vi "patientTrainingView.vi"() -> ()   [LabVIEW 2019]
doc: "40"
uses:
  03_Home/controller/logoutBtn.ctl
  03_Home/controller/exitBtn.ctl
  <vilib>/Utility/miscctls.llb/LVPointTypeDef.ctl
  subVI/patients_state.ctl
  <vilib>/Utility/miscctls.llb/LVSelectionTypeDef.ctl
  03_Home/controller/pannelState.ctl
  globalValue.vi
panel:
  out "patients_nm2":string
  out "training_id":string[](array[string])
  out "totalCount":string
  out "patients_info":string
  out "patients_notes":string
  out "patients_nm":string
  out "patients_id":string
  in  "patients_weight":dbl format="%.1f kg"
  in  "patients_age":dbl
  in  "patients_height":dbl format="%.1f cm"
  out "patients_birthdate":dbl format="%<%Y.%m.%d.>T"
  in  "backPage":bool
  in  "btnGroup":T1
  out "totalPage":i8
  out "crrentPage":i8
  in  "leftBtn":bool
  in  "rightBtn":bool
  in  "patientList":i32(listbox)
  in  "cancelBtn":bool
  in  "updateBtn":bool
  in  "deleteBtn":bool
  out "userDetailInfo":string[](array[string])
  in  "Help Button":bool
  in  "LogOut Button":T2
  in  "Exit Button":T3
  out "userNm":string
  # "/"
  # "|"
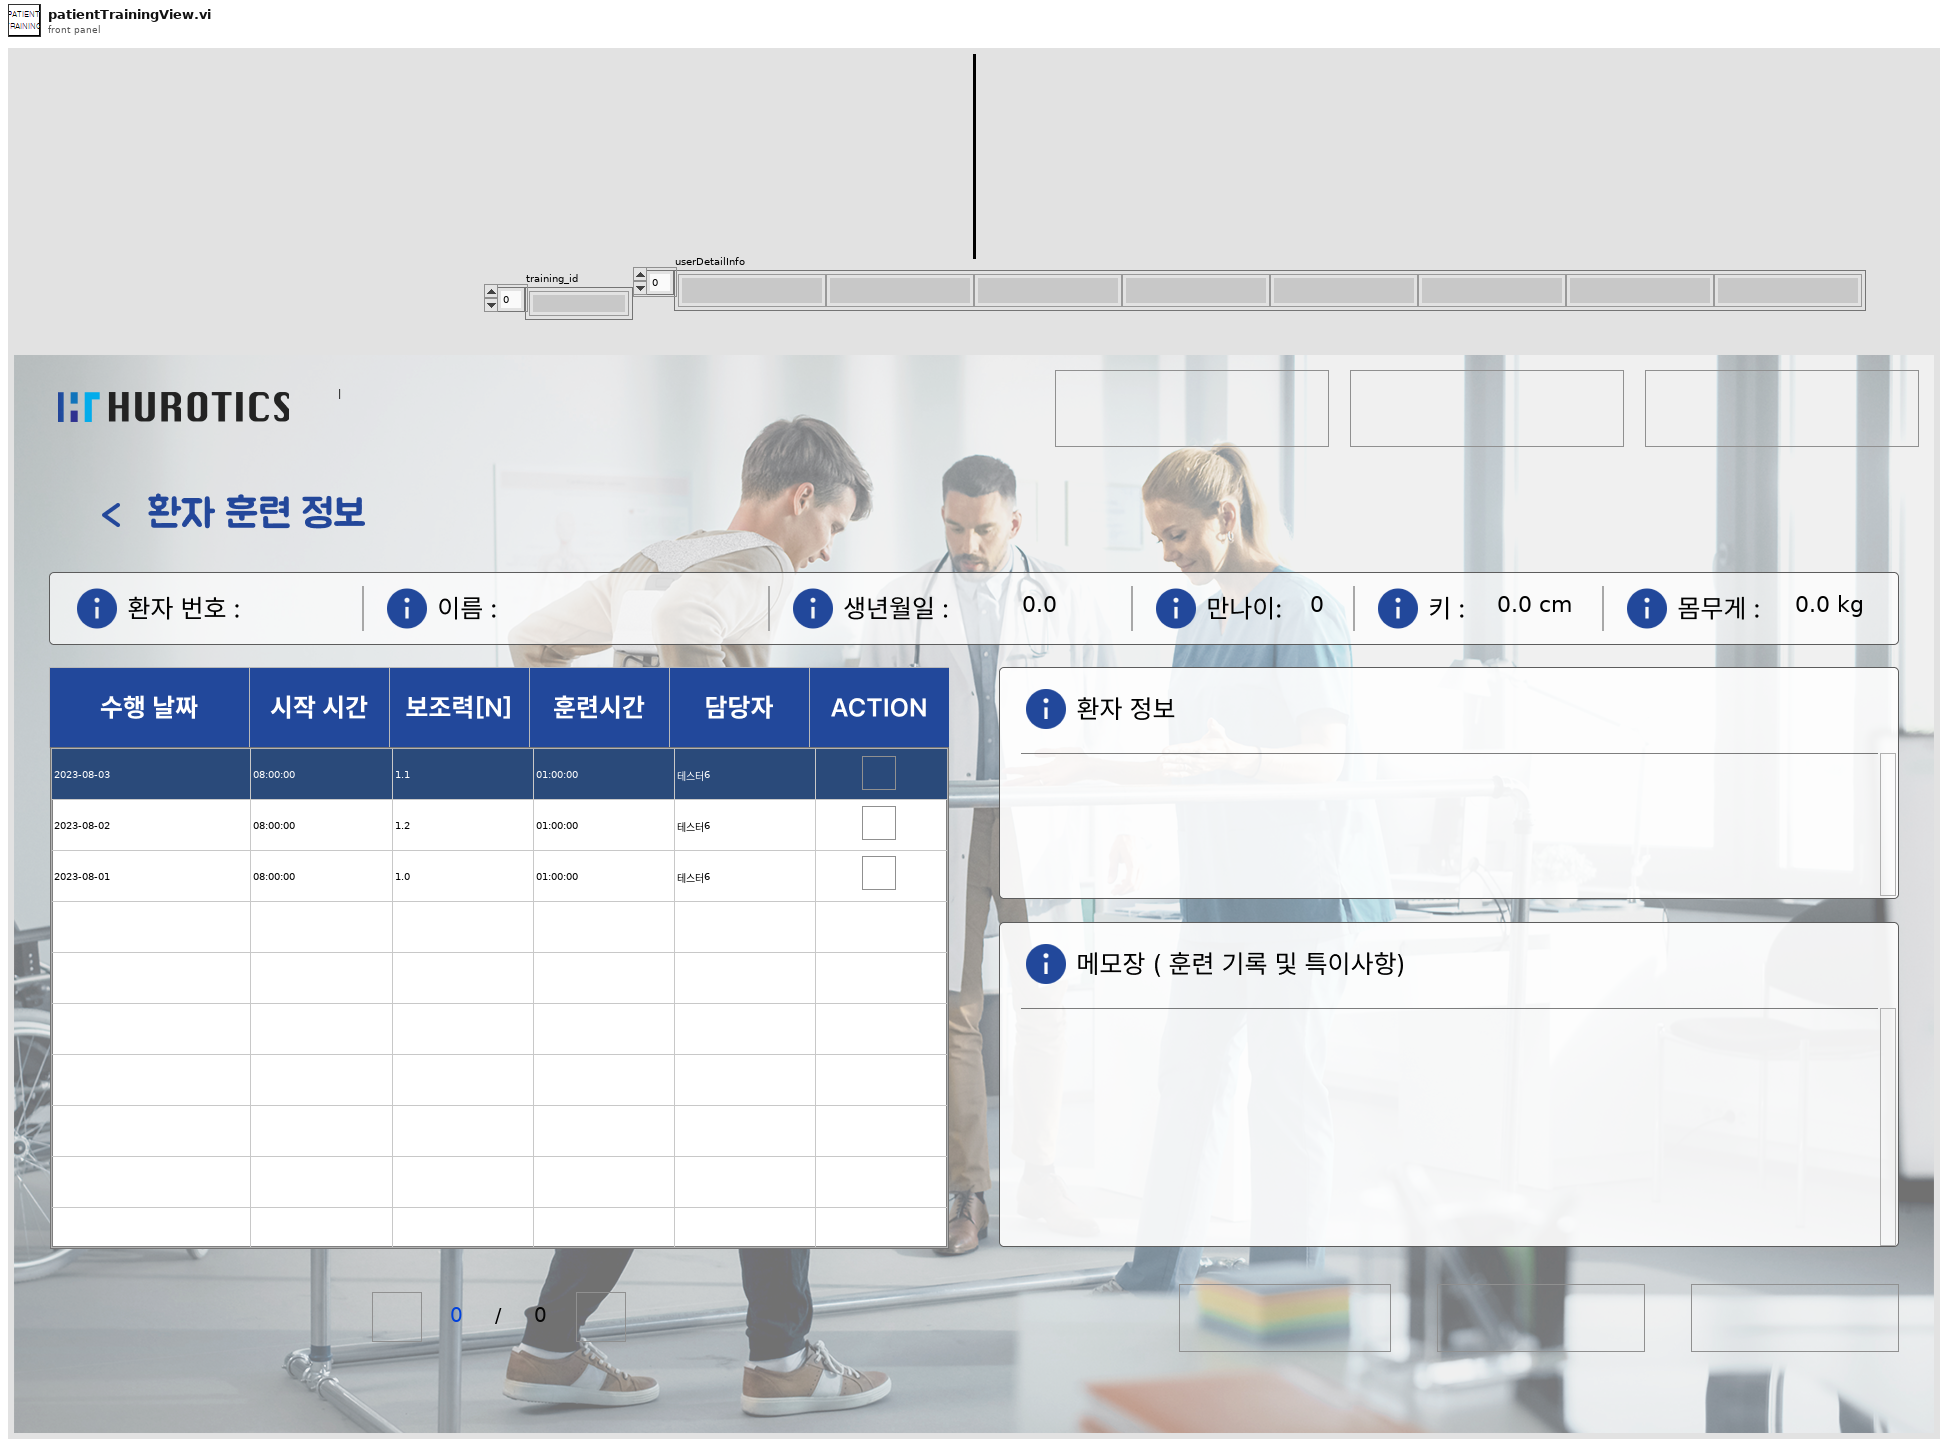
[diagram p1: front panel]
types:
  T1 = cluster{"detailBtn":bool, "detailBtn":bool, "detailBtn 2":bool, "detailBtn 3":bool, "detailBtn 4":bool, "detailBtn 5":bool, "detailBtn 6":bool, "detailBtn 7":bool, "detailBtn 8":bool, "detailBtn 9":bool}
  T2 = typedef "logoutBtn.ctl" = bool
  T3 = typedef "exitBtn.ctl" = bool
  T4 = typedef "LVPointTypeDef.ctl" = cluster{"Horizontal":i16, "Vertical":i16}
  T5 = typedef "patients_state.ctl" = enum16{"connection", "create", "getReadList", "getRead", "getCount", "update", "delete", "trash", "restore", "close"}
  T6 = enum16{"connection", "create", "getReadList", "getRead", "getCount", "update", "delete", "close"}
  T7 = typedef "LVSelectionTypeDef.ctl" = cluster{"Selection Start":u32, "Selection End":u32}
  T8 = enum8{"Enabled", "Disabled", "Disabled and Grayed Out"}
  T9 = typedef "pannelState.ctl" = enum16{"Init", "LogIn", "SignUpView", "Home", "Management_patientList", "Management_patientTrashtList", "Management_patientCreate", "Management_patientUpdate", "Management_patientTraining", "Management_patientTrainingDetail", "H-MEDI PatientList", "H-MEDI HardwareCtl", "Adjust", "FineTuning", "UserList", "UserDetail", "Exit"}
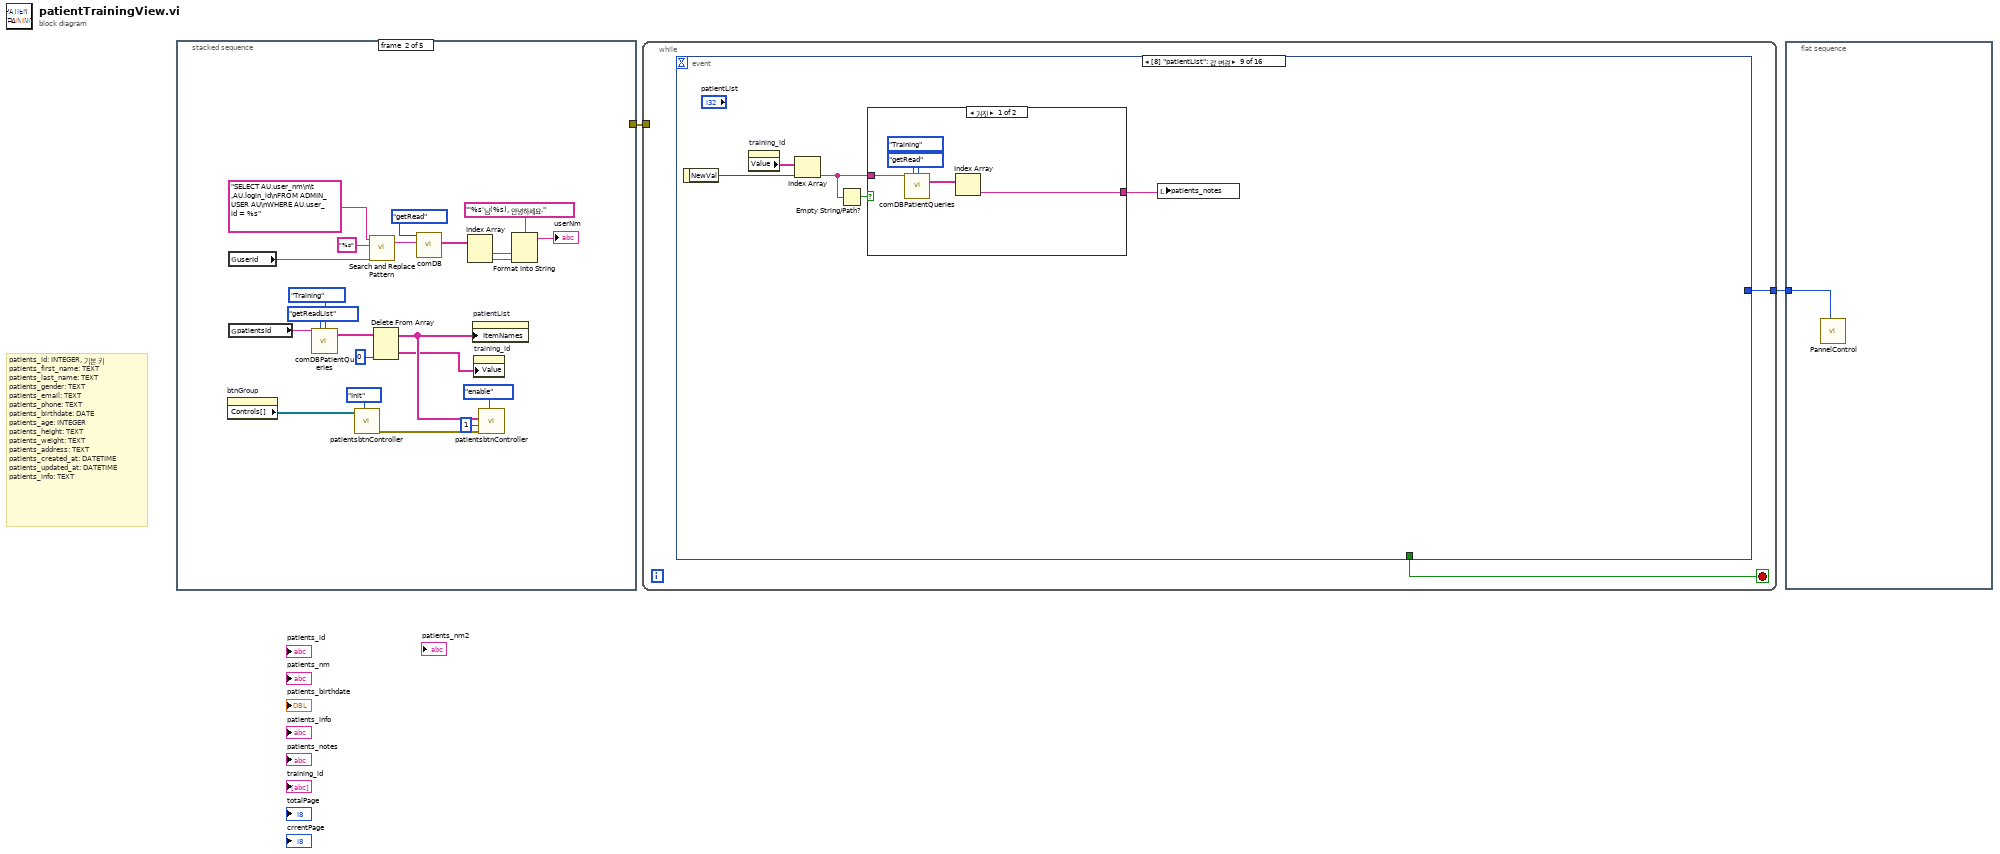
[diagram p0: block diagram]
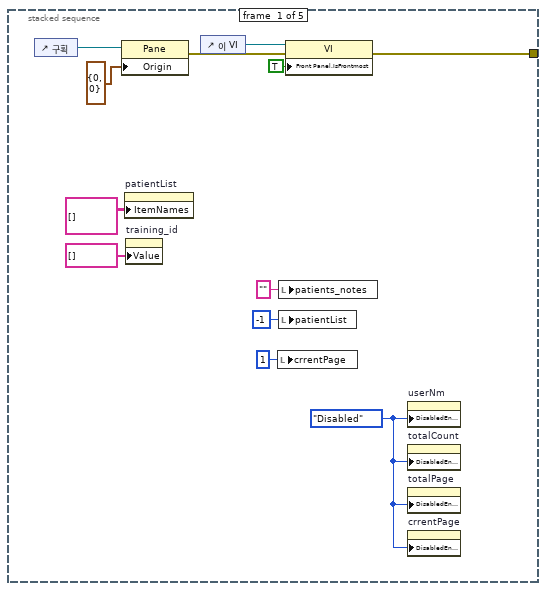
[diagram p2: hidden frame]
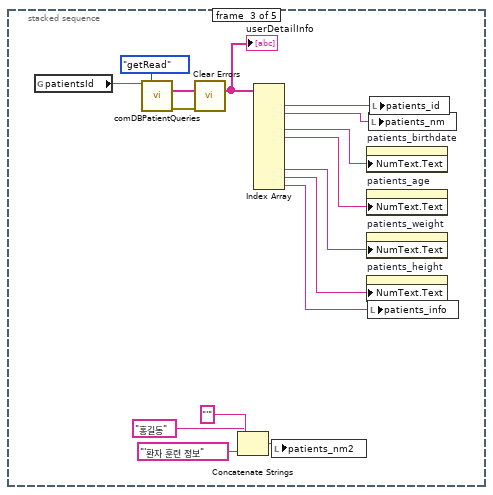
[diagram p3: hidden frame]
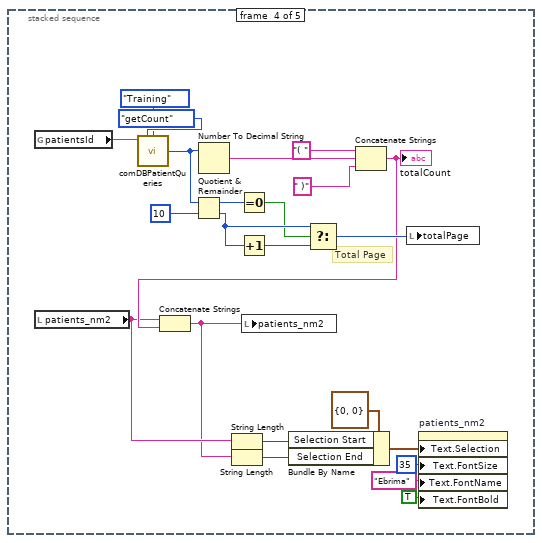
[diagram p4: hidden frame]
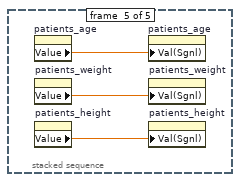
[diagram p5: hidden frame]
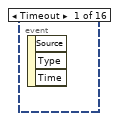
[diagram p6: hidden frame]
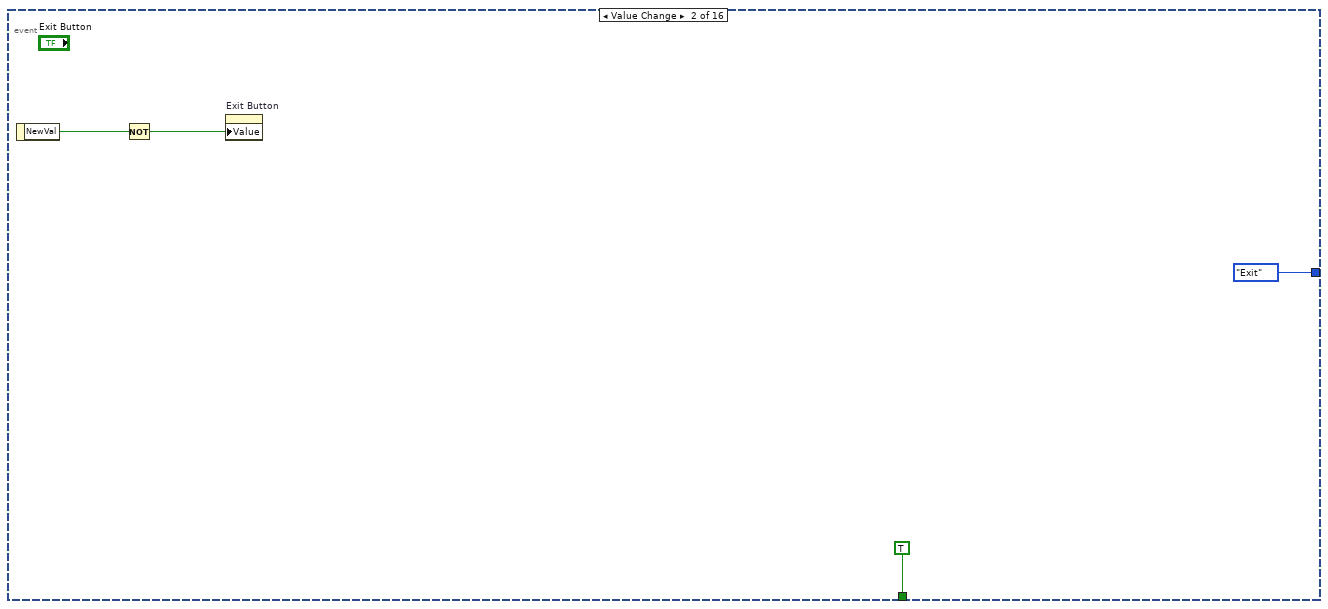
[diagram p7: hidden frame]
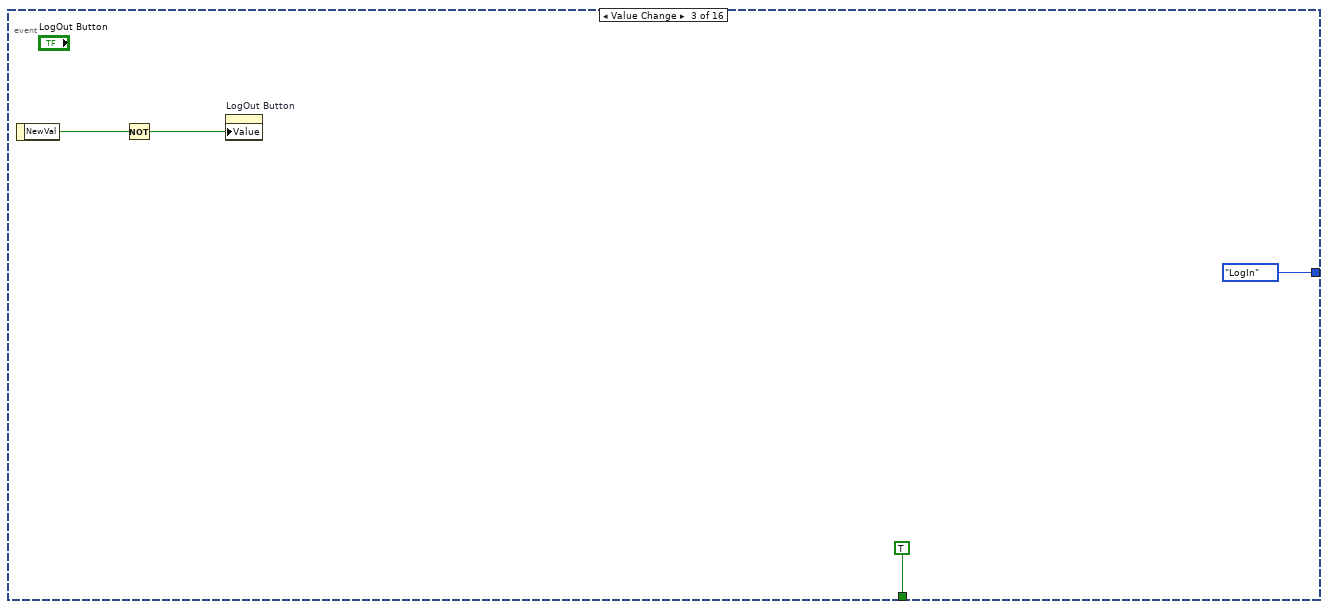
[diagram p8: hidden frame]
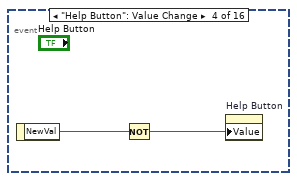
[diagram p9: hidden frame]
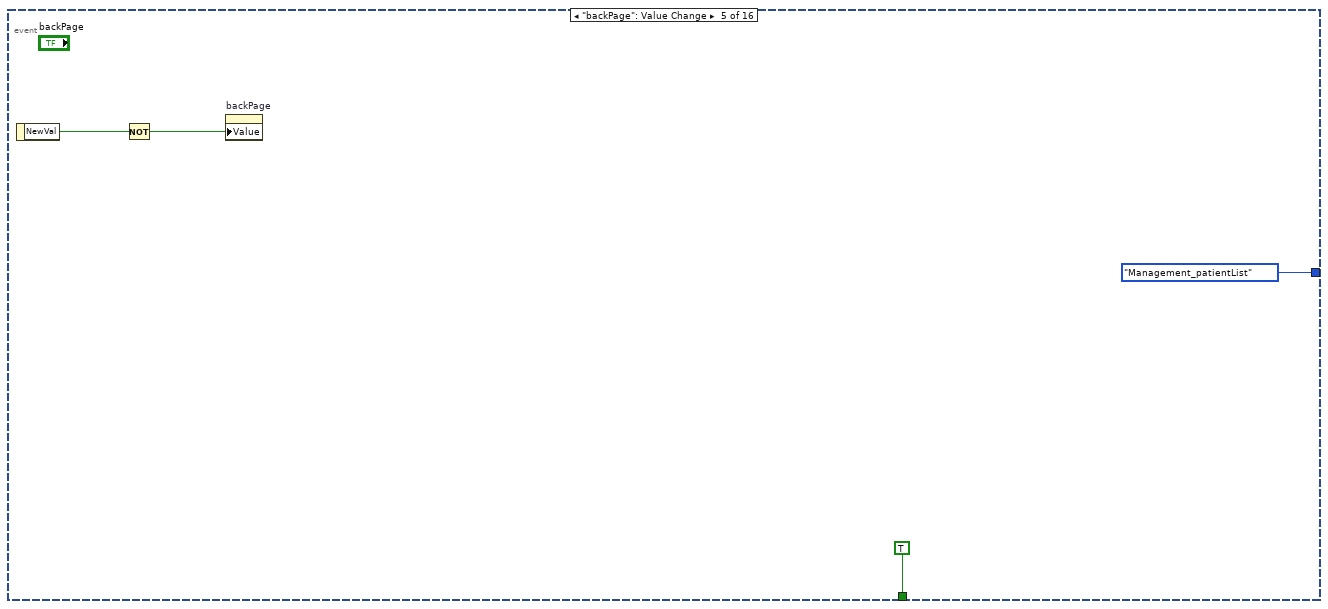
[diagram p10: hidden frame]
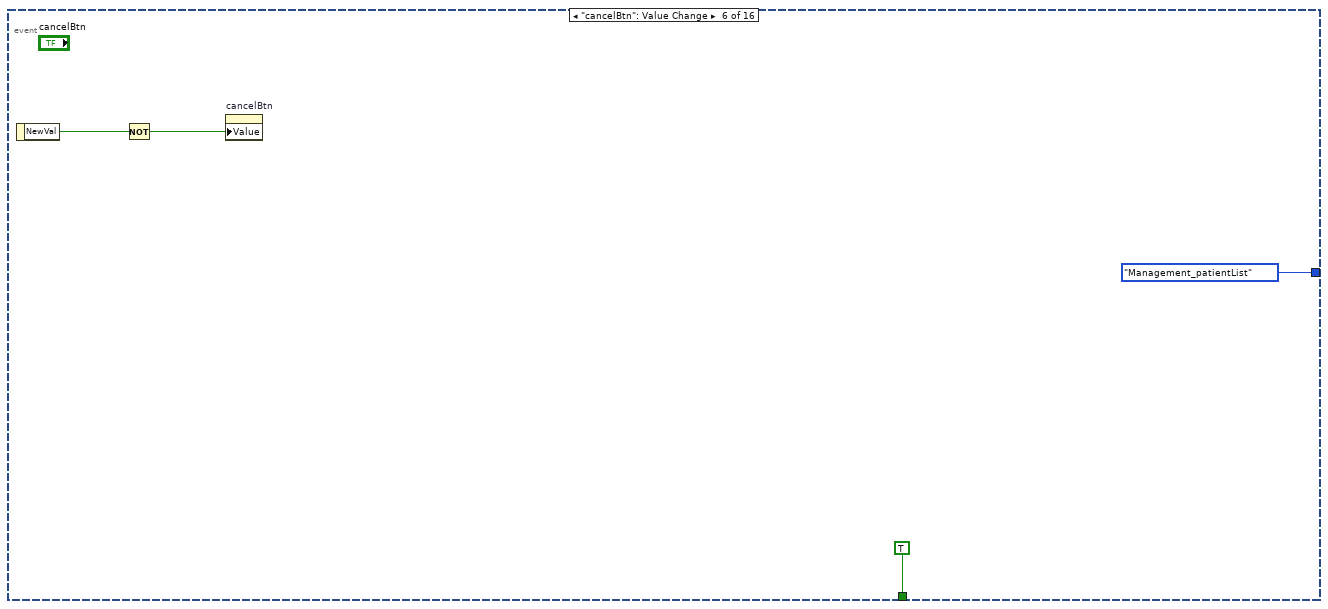
[diagram p11: hidden frame]
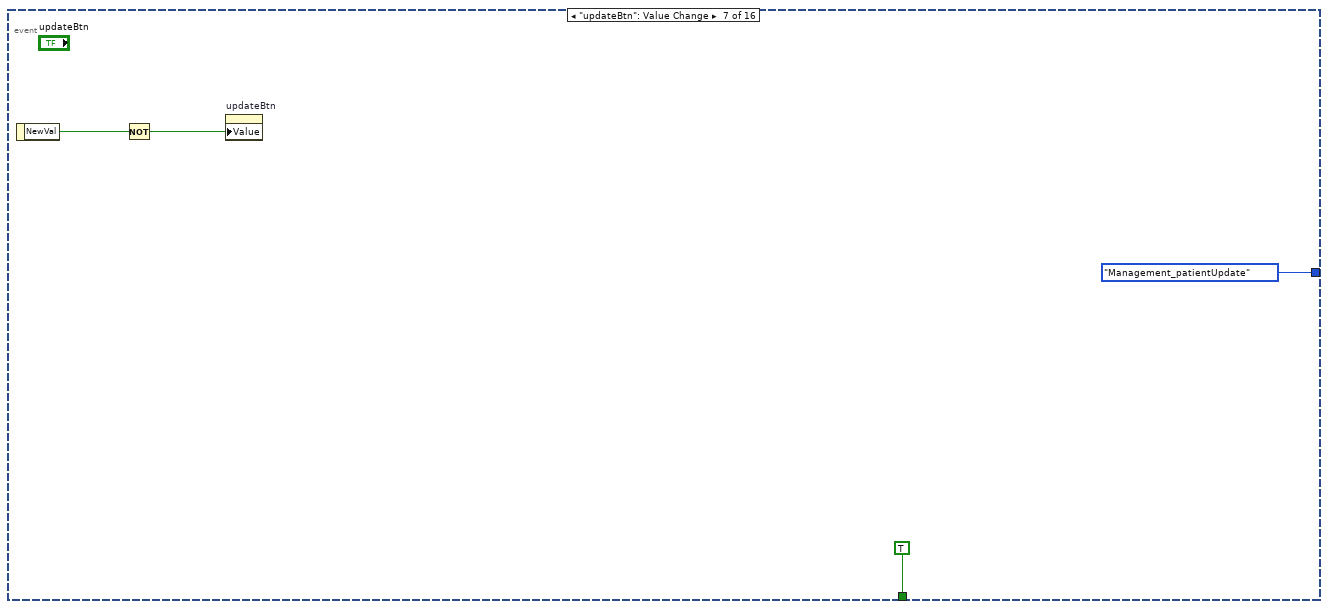
[diagram p12: hidden frame]
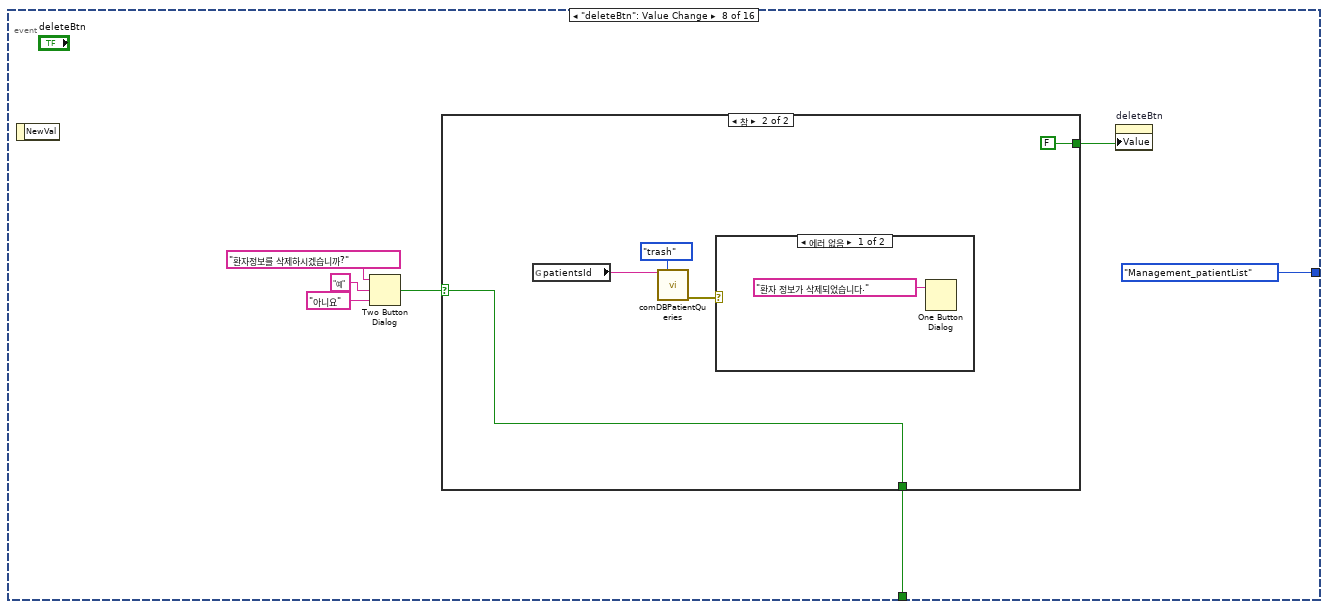
[diagram p13: hidden frame]
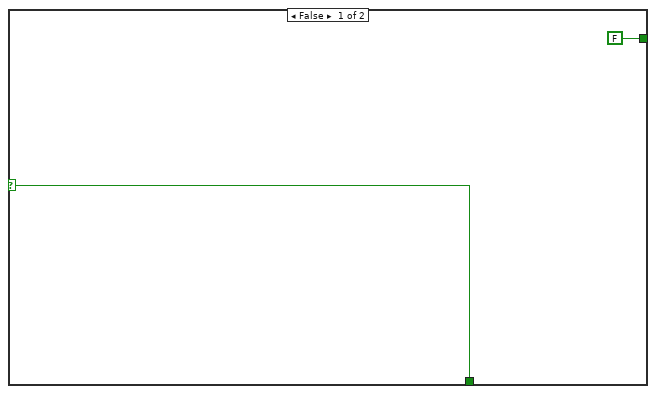
[diagram p14: hidden frame]
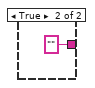
[diagram p16: hidden frame]
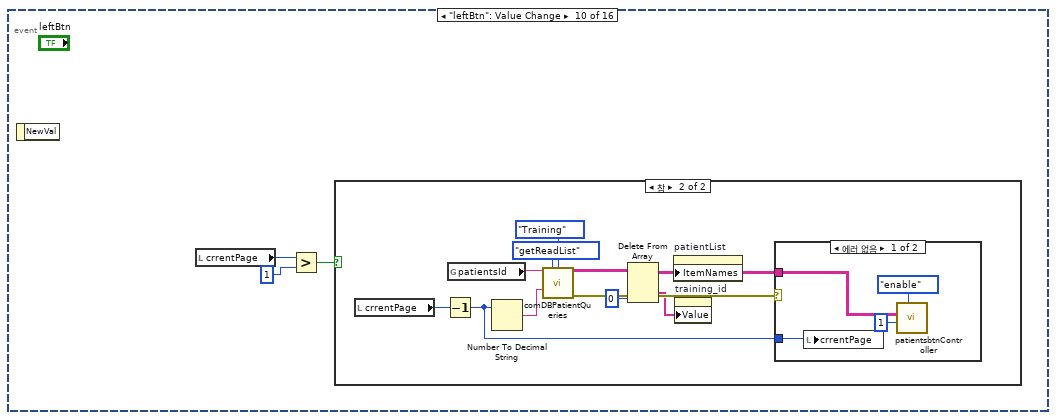
[diagram p17: hidden frame]
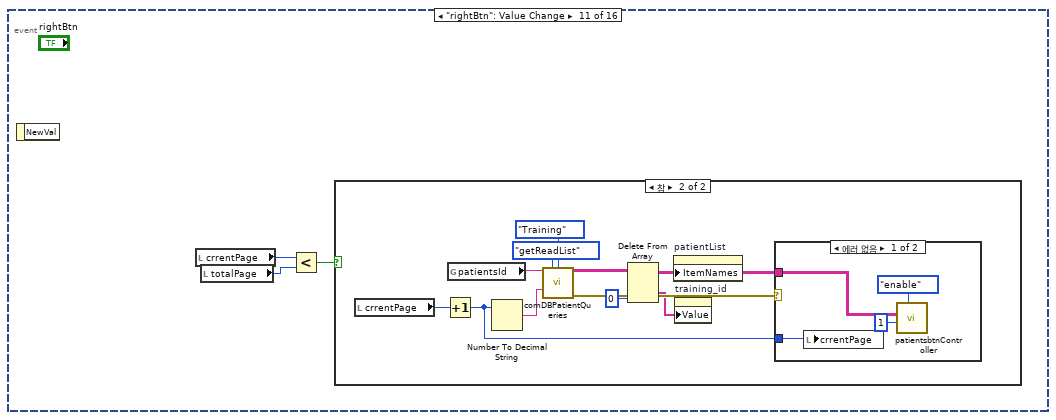
[diagram p20: hidden frame]
diagram:
  # "patients_id: INTEGER, 기본 키\npatients_first_name: TEXT\npatients_last_name: TEXT\npatients_gender: TEXT\npatients_email: TEXT\npatients_phone: TEXT\npatients_birthdate: DATE\npatients_age: INTEGER\npatients_height: TEXT\npatients_weight: TEXT\npatients_address: TEXT\npatients_created_at: DATETIME\npatients_updated_at: DATETIME\npatients_info: TEXT"
  n1 = stacked-sequence {
    tunnel: [w9 _ _ _ _] -> w1
    frame #0 {
      w7 = T8."Disabled" ("비활성화")
      n2 = control-ref of="구획"() -> (w12:refnum<vi>)
      n3 = property class="Pane"(reference=w12, "Origin"=T4 {"Horizontal"=0, "Vertical"=0} ("원점")) -> (error out=w10:errorcluster)  [unwired: 1 in, 1 out]
      n4 = property on="patientList" class="MCListbox (엄격한)"("ItemNames"=string[][] [] ("아이템 이름")) -> ()  [unwired: 2 in, 2 out]
      n5 = property on="training_id" class="Arr (엄격한)"("Value"=string[] [] ("training_id")) -> ()  [unwired: 2 in, 2 out]
      n6 = control-ref of="이 VI"() -> (w14:refnum<vi>)
      n7 = local write "crrentPage"(i8 1 ("crrentPage")) -> ()
      n8 = local write "patients_notes"("" ("patients_notes")) -> ()
      n9 = local write "patientList"(-1 ("patientList")) -> ()
      n10 = property class="VI"(reference=w14, error in=w10, "Front Panel.IsFrontmost"=TRUE ("프런트패널 윈도우:맨 앞으로")) -> (error out=w9:errorcluster)  [unwired: 1 out]
      n11 = property on="userNm" class="Str"("DisabledEnum"=w7) -> ()  [unwired: 2 in, 2 out]
      n12 = property on="totalCount" class="Str"("DisabledEnum"=w7) -> ()  [unwired: 2 in, 2 out]
      n13 = property on="totalPage" class="DigNum (엄격한)"("DisabledEnum"=w7) -> ()  [unwired: 2 in, 2 out]
      n14 = property on="crrentPage" class="DigNum (엄격한)"("DisabledEnum"=w7) -> ()  [unwired: 2 in, 2 out]
    }
    frame #1 {
      n15 = property on="btnGroup" class="Clust"() -> ("Controls[]"=w21:refnum<vi>[])  [unwired: 2 in, 2 out]
      n16 = global read "globalValue.vi" "userId"() -> (w27:string)
      n17 = global read "globalValue.vi" "patientsId"() -> (w16:string)
      n18 = call "comDBPatientQueries.vi"("id"=w16, "State"=patients_state."getReadList", "select"=enum16{"Default", "Trash", "Training"}."Training") -> ("resultList"=w20:string[][])  [unwired: 9 in, 3 out]
      n19 = call "patientsbtnController.vi"("state"=enum16{"Init", "disable", "enable"}."Init", "Controls[]"=w21) -> ("error out"=w25:errorcluster)  [unwired: 9 in]
      n20 = call <vilib>:"Search and Replace Pattern.vi"("string"="SELECT AU.user_nm\n\t         ,AU.login_id\nFROM ADMIN_USER AU\nWHERE AU.user_id = %s" ("Query"), "regular expression (\"\")"="%s" ("regular expression (\"\")"), "replace string (\"\")"=w27) -> ("result string"=w28:string)  [unwired: 2 in, 1 out]
      n21 = Delete From Array(array=w20, index (col)=0 ("비활성화된 인덱스 (열)")) -> (deleted portion=w17:string[], array with subset deleted=w18:string[][])  [unwired: 2 in]
      n22 = call "comDB.vi"("Query"=w28, "State"=T6."getRead") -> ("result1DArray"=w34:string[])  [unwired: 5 in, 3 out]
      n23 = Index Array(array=w34) -> (element #1=w33:string, element #2=w32:string)  [unwired: 2 in]
      n24 = property on="patientList" class="MCListbox (엄격한)"("ItemNames"=w18) -> ()  [unwired: 2 in, 2 out]
      n25 = property on="training_id" class="Arr (엄격한)"("Value"=w17) -> ()  [unwired: 2 in, 2 out]
      n26 = call "patientsbtnController.vi"("state"=enum16{"Init", "disable", "enable"}."enable", "error in (no error)"=w25, "버튼개수"=1, "2dArray"=w18) -> ()  [unwired: 7 in, 1 out]
      n27 = Format Into String(format string="'%s'님(%s), 안녕하세요." ("문자열"), w33, w32) -> (resulting string=→"userNm":string)  [unwired: 2 in, 1 out]
    }
    frame #2 {
      n28 = global read "globalValue.vi" "patientsId"() -> (w46:string)
      n29 = call "comDBPatientQueries.vi"("id"=w46, "State"=patients_state."getRead") -> ("result1DArray"=w51:string[], "error out"=w50:errorcluster)  [unwired: 10 in, 2 out]
      "userDetailInfo" <- w51
      n30 = call <vilib>:"Clear Errors.vi"("error in (no error)"=w50) -> ()  [unwired: 5 in, 2 out]
      n31 = Concatenate Strings("'" ("문자열"), "홍길동" ("문자열"), "'환자 훈련 정보" ("문자열")) -> (w40:string)
      n32 = Index Array(array=w51) -> (element #1=w48:string, element #2=w47:string, element #4=w45:string, element #5=w44:string, element #9=w43:string, element #10=w42:string, element #11=w41:string)  [unwired: 11 in, 4 out]
      n33 = local write "patients_nm2"(w40) -> ()
      n34 = property on="patients_birthdate" class="DigNum (엄격한)"("NumText.Text"=w45) -> ()  [unwired: 2 in, 2 out]
      n35 = property on="patients_age" class="DigNum (엄격한)"("NumText.Text"=w44) -> ()  [unwired: 2 in, 2 out]
      n36 = property on="patients_weight" class="DigNum (엄격한)"("NumText.Text"=w43) -> ()  [unwired: 2 in, 2 out]
      n37 = property on="patients_height" class="DigNum (엄격한)"("NumText.Text"=w42) -> ()  [unwired: 2 in, 2 out]
      n38 = local write "patients_info"(w41) -> ()
      n39 = local write "patients_nm"(w47) -> ()
      n40 = local write "patients_id"(w48) -> ()
    }
    frame #3 {
      # "Total Page"
      n41 = global read "globalValue.vi" "patientsId"() -> (w62:string)
      n42 = local read "patients_nm2"() -> (w53:string)
      n43 = call "comDBPatientQueries.vi"("id"=w62, "State"=patients_state."getCount", "select"=enum16{"Default", "Trash", "Training"}."Training") -> ("count"=w74:i64)  [unwired: 9 in, 3 out]
      n44 = Quotient & Remainder(x=w74, y=i64 10) -> (x-y*floor(x/y)=w72:i64, floor(x/y)=w73:i64)
      n45 = Number To Decimal String(number=w74) -> (decimal integer string=w69:string)  [unwired: 1 in]
      n46 = String Length(string=w53) -> (length=w60:i32)
      n47 = Equal To 0?(x=w72) -> (x = 0?=w71:bool)
      n48 = Increment(x=w73) -> (x+1=w70:i64)
      n49 = Select(t=w73, s=w71, f=w70) -> (s? t:f=w64:i64)
      n50 = Concatenate Strings("( ", w69, " )") -> (w55:string)
      "totalCount" <- w55
      n51 = Concatenate Strings(w53, w55) -> (w52:string)
      n52 = String Length(string=w52) -> (length=w54:i32)
      n53 = local write "patients_nm2"(w52) -> ()
      n54 = Bundle By Name(cluster=T7 {"Selection Start"=0, "Selection End"=0} ("텍스트.선택"), "Selection Start"=w60, "Selection End"=w54) -> (w59:T7)
      n55 = local write "totalPage"(w64) -> ()
      n56 = property on="patients_nm2" class="Str"("Text.Selection"=w59, "Text.FontSize"=u32 35 ("텍스트.폰트:크기"), "Text.FontName"="Ebrima" ("텍스트.폰트:이름"), "Text.FontBold"=TRUE ("텍스트.폰트:굵은체")) -> ()  [unwired: 2 in, 2 out]
    }
    frame #4 {
      n57 = property on="patients_age" class="DigNum (엄격한)"() -> ("Value"=w77:dbl)  [unwired: 2 in, 2 out]
      n58 = property on="patients_weight" class="DigNum (엄격한)"() -> ("Value"=w76:dbl)  [unwired: 2 in, 2 out]
      n59 = property on="patients_height" class="DigNum (엄격한)"() -> ("Value"=w75:dbl)  [unwired: 2 in, 2 out]
      n60 = property on="patients_age" class="DigNum (엄격한)"("Val(Sgnl)"=w77) -> ()  [unwired: 2 in, 2 out]
      n61 = property on="patients_weight" class="DigNum (엄격한)"("Val(Sgnl)"=w76) -> ()  [unwired: 2 in, 2 out]
      n62 = property on="patients_height" class="DigNum (엄격한)"("Val(Sgnl)"=w75) -> ()  [unwired: 2 in, 2 out]
    }
  }
  n63 = while {
    tunnel: [w78] -> w2
    tunnel: w1 -> [_]
    stop <- w79 stop-if-true
    n64 = event shown="[8] \"patientList\": 값 변경" {
      selector: _ -> [_ _ _ _ _ _ _ _ _ _ _ _ _ _ _ _]
      dyn-events: _ -> [_ _ _ _ _ _ _ _ _ _ _ _ _ _ _ _]
      timeout: _ -> [_ _ _ _ _ _ _ _ _ _ _ _ _ _ _ _]
      tunnel: [_ TRUE TRUE _ TRUE TRUE TRUE w103 _ _ _ TRUE w173 _ _ _] -> w79
      tunnel: [_ pannelState."Exit" ("State") pannelState."LogIn" ("State") _ pannelState."Management_patientList" ("State") pannelState."Management_patientList" ("State") pannelState."Management_patientUpdate" ("State") pannelState."Management_patientList" ("State") _ _ _ pannelState."Management_patientTrainingDetail" ("State") pannelState."Management_patientTrainingDetail" ("State") _ _ _] -> w78
      event Timeout {
        n65 = event-data() -> ()  [unwired: 1 in, 3 out]
      }
      event Value Change {
        n66 = event-data() -> ("NewVal"=w81:T3)  [unwired: 1 in]
        n67 = Not(x=w81) -> (.not. x?=w80:T3)
        n68 = property on="Exit Button" class="Bool (엄격한)"("Value"=w80) -> ()  [unwired: 2 in, 2 out]
      }
      event Value Change {
        n69 = event-data() -> ("NewVal"=w85:T2)  [unwired: 1 in]
        n70 = Not(x=w85) -> (.not. x?=w84:T2)
        n71 = property on="LogOut Button" class="Bool (엄격한)"("Value"=w84) -> ()  [unwired: 2 in, 2 out]
      }
      event "Help Button": Value Change {
        n72 = event-data() -> ("NewVal"=w89:bool)  [unwired: 1 in]
        n73 = Not(x=w89) -> (.not. x?=w88:bool)
        n74 = property on="Help Button" class="Bool (엄격한)"("Value"=w88) -> ()  [unwired: 2 in, 2 out]
      }
      event "backPage": Value Change {
        n75 = event-data() -> ("NewVal"=w92:bool)  [unwired: 1 in]
        n76 = Not(x=w92) -> (.not. x?=w91:bool)
        n77 = property on="backPage" class="Bool (엄격한)"("Value"=w91) -> ()  [unwired: 2 in, 2 out]
      }
      event "cancelBtn": Value Change {
        n78 = event-data() -> ("NewVal"=w97:bool)  [unwired: 1 in]
        n79 = Not(x=w97) -> (.not. x?=w95:bool)
        n80 = property on="cancelBtn" class="Bool (엄격한)"("Value"=w95) -> ()  [unwired: 2 in, 2 out]
      }
      event "updateBtn": Value Change {
        n81 = event-data() -> ("NewVal"=w99:bool)  [unwired: 1 in]
        n82 = Not(x=w99) -> (.not. x?=w98:bool)
        n83 = property on="updateBtn" class="Bool (엄격한)"("Value"=w98) -> ()  [unwired: 2 in, 2 out]
      }
      event "deleteBtn": Value Change {
        n84 = event-data() -> ()  [unwired: 1 in, 1 out]
        n85 = Two Button Dialog(message="환자정보를 삭제하시겠습니까?" ("메시지"), 1:"아니요" ("거짓 버튼 이름(\"취소\")"), 2:"예" ("참 버튼 이름(\"확인\")")) -> (T button?=w105:bool)
        n86 = case shown="참" w105 {
          selector: w105 -> [w109 w112]
          tunnel: [FALSE ("deleteBtn") FALSE ("deleteBtn")] -> w104
          tunnel: [w109 w112] -> w103
          frame False {
          }
          frame True {
            n87 = global read "globalValue.vi" "patientsId"() -> (w111:string)
            n88 = call "comDBPatientQueries.vi"("id"=w111, "State"=patients_state."trash") -> ("error out"=w115:errorcluster)  [unwired: 10 in, 3 out]
            n89 = case shown="에러 없음" w115 {
              frame No Error {
                n90 = One Button Dialog(message="환자 정보가 삭제되었습니다." ("메시지")) -> ()  [unwired: 1 in, 1 out]
              }
              frame Error {
              }
            }
          }
        }
        n91 = property on="deleteBtn" class="Bool (엄격한)"("Value"=w104) -> ()  [unwired: 2 in, 2 out]
      }
      event "patientList": Value Change {
        n92 = event-data() -> ("NewVal"=w120:i32)  [unwired: 1 in]
        n93 = property on="training_id" class="Arr (엄격한)"() -> ("Value"=w121:string[])  [unwired: 2 in, 2 out]
        n94 = Index Array(array=w121, index=w120) -> (element=w119:string)
        n95 = Empty String/Path?(string/path=w119) -> (empty?=w118:bool)
        n96 = case shown="거짓" w118 {
          tunnel: w119 -> [w123 _]
          tunnel: [w122 "" ("Text")] -> w117
          frame False {
            n97 = call "comDBPatientQueries.vi"("id"=w123, "State"=patients_state."getRead", "select"=enum16{"Default", "Trash", "Training"}."Training") -> ("result1DArray"=w124:string[])  [unwired: 9 in, 3 out]
            n98 = Index Array(array=w124) -> (element=w122:string)  [unwired: 1 in]
          }
          frame True {
          }
        }
        n99 = local write "patients_notes"(w117) -> ()
      }
      event "leftBtn": Value Change {
        n100 = event-data() -> ()  [unwired: 1 in, 1 out]
        n101 = local read "crrentPage"() -> (w130:i8)
        n102 = Greater?(x=w130, y=1) -> (0:w129:bool)
        n103 = case shown="참" w129 {
          frame False {
          }
          frame True {
            n104 = local read "crrentPage"() -> (w137:i8)
            n105 = Decrement(x=w137) -> (x-1=w141:i8)
            n106 = global read "globalValue.vi" "patientsId"() -> (w131:string)
            n107 = Number To Decimal String(number=w141) -> (decimal integer string=w139:string)  [unwired: 1 in]
            n108 = call "comDBPatientQueries.vi"("id"=w131, "State"=patients_state."getReadList", "select"=enum16{"Default", "Trash", "Training"}."Training", "crrentPage"=w139) -> ("resultList"=w134:string[][], "error out"=w138:errorcluster)  [unwired: 8 in, 2 out]
            n109 = Delete From Array(array=w134, index (col)=0 ("비활성화된 인덱스 (열)")) -> (deleted portion=w132:string[], array with subset deleted=w133:string[][])  [unwired: 2 in]
            n110 = property on="patientList" class="MCListbox (엄격한)"("ItemNames"=w133) -> ()  [unwired: 2 in, 2 out]
            n111 = property on="training_id" class="Arr (엄격한)"("Value"=w132) -> ()  [unwired: 2 in, 2 out]
            n112 = case shown="에러 없음" w138 {
              tunnel: w141 -> [w143 _]
              tunnel: w133 -> [w144 _]
              frame No Error {
                n113 = local write "crrentPage"(w143) -> ()
                n114 = call "patientsbtnController.vi"("state"=enum16{"Init", "disable", "enable"}."enable", "버튼개수"=1, "2dArray"=w144) -> ()  [unwired: 8 in, 1 out]
              }
              frame Error {
              }
            }
          }
        }
      }
      event "rightBtn": Value Change {
        n115 = event-data() -> ()  [unwired: 1 in, 1 out]
        n116 = local read "crrentPage"() -> (w148:i8)
        n117 = local read "totalPage"() -> (w146:i8)
        n118 = Less?(x=w148, y=w146) -> (x < y?=w147:bool)
        n119 = case shown="참" w147 {
          frame False {
          }
          frame True {
            n120 = local read "crrentPage"() -> (w155:i8)
            n121 = Increment(x=w155) -> (x+1=w159:i8)
            n122 = global read "globalValue.vi" "patientsId"() -> (w149:string)
            n123 = Number To Decimal String(number=w159) -> (decimal integer string=w157:string)  [unwired: 1 in]
            n124 = call "comDBPatientQueries.vi"("id"=w149, "State"=patients_state."getReadList", "select"=enum16{"Default", "Trash", "Training"}."Training", "crrentPage"=w157) -> ("resultList"=w152:string[][], "error out"=w156:errorcluster)  [unwired: 8 in, 2 out]
            n125 = Delete From Array(array=w152, index (col)=0 ("비활성화된 인덱스 (열)")) -> (deleted portion=w150:string[], array with subset deleted=w151:string[][])  [unwired: 2 in]
            n126 = property on="patientList" class="MCListbox (엄격한)"("ItemNames"=w151) -> ()  [unwired: 2 in, 2 out]
            n127 = property on="training_id" class="Arr (엄격한)"("Value"=w150) -> ()  [unwired: 2 in, 2 out]
            n128 = case shown="에러 없음" w156 {
              tunnel: w159 -> [w161 _]
              tunnel: w151 -> [w162 _]
              frame No Error {
                n129 = local write "crrentPage"(w161) -> ()
                n130 = call "patientsbtnController.vi"("state"=enum16{"Init", "disable", "enable"}."enable", "버튼개수"=1, "2dArray"=w162) -> ()  [unwired: 8 in, 1 out]
              }
              frame Error {
              }
            }
          }
        }
      }
      event "btnGroup": Value Change {
        n131 = event-data() -> ("NewVal"=w169:T1)  [unwired: 1 in]
        n132 = Cluster To Array(cluster=w169) -> (array=w171:bool[])
        n133 = Search 1D Array(1D array=w171, element=TRUE ("원소")) -> (index of element=w168:i32)  [unwired: 1 in]
        n134 = property on="training_id" class="Arr (엄격한)"() -> ("Value"=w167:string[])  [unwired: 2 in, 2 out]
        n135 = Index Array(array=w167, index=w168) -> (element=w164:string)
        n136 = global write "globalValue.vi" "traningId"(w164) -> ()
      }
      event "patientList": Double Click {
        n137 = event-data() -> ("Row"=w176:i32)  [unwired: 1 in]
        n138 = property on="training_id" class="Arr (엄격한)"() -> ("Value"=w177:string[])  [unwired: 2 in, 2 out]
        n139 = Index Array(array=w177, index=w176) -> (element=w174:string)
        n140 = Empty String/Path?(string/path=w174) -> (empty?=w175:bool)
        n141 = case shown="거짓" w175 {
          tunnel: w174 -> [w179 _]
          tunnel: [TRUE _] -> w173
          frame False {
            n142 = global write "globalValue.vi" "traningId"(w179) -> ()
          }
          frame True {
          }
        }
      }
      event "patients_age": Value Change; "patients_age": Mouse Down {
        n143 = event-data() -> ("CtlRef"=w180:refnum<vi>)  [unwired: 1 in]
        n144 = call "textColor.vi"("디지털 입력"=w180) -> ()  [unwired: 11 in]
      }
      event "patients_weight": Value Change; "patients_weight": Mouse Down {
        n145 = event-data() -> ("CtlRef"=w181:refnum<vi>)  [unwired: 1 in]
        n146 = call "textColor.vi"("디지털 입력"=w181) -> ()  [unwired: 11 in]
      }
      event "patients_height": Value Change; "patients_height": Mouse Down {
        n147 = event-data() -> ("CtlRef"=w182:refnum<vi>)  [unwired: 1 in]
        n148 = call "textColor.vi"("디지털 입력"=w182) -> ()  [unwired: 11 in]
      }
    }
  }
  n149 = flat-sequence {
    tunnel: w2 -> [w183]
    frame #0 {
      n150 = call "PannelControl.vi"("State"=w183) -> ()  [unwired: 10 in, 1 out]
    }
  }
